vi "RSZVB Set Frequency Conversion Source.vi"(8 "error in (no error)":errorcluster {"code" format="%.0x"}, 10 "Conversion Source (0: Meas. at Source Frequency)":i32(ring) items=["Measurement at Source Frequency", "Measurement at Receiver Frequency"], 11 "VISA session":refnum<visa-resource-name>) -> (0 "error out":errorcluster {"code" format="%.0x"}, 3 "dup VISA session":refnum<visa-resource-name>)   [LabVIEW 2011]
doc: "This VI selects the test setup (internal or external sources) for the frequency converter measurement (with option ZVA-K8, Enhanced Frequency Conversion). \n\n\nNote(s):\n\n(1) This VI is available only on R&S ZVA and ZVT instrument.\n\nRemote-control command(s):\nSENSe<Ch>:FREQuency:CONVersion:DEVice:MODE RILI | RILE"
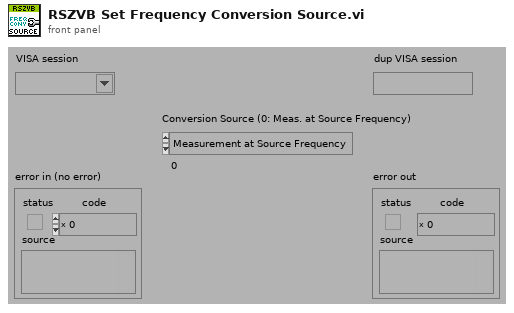
[diagram p1: front panel]
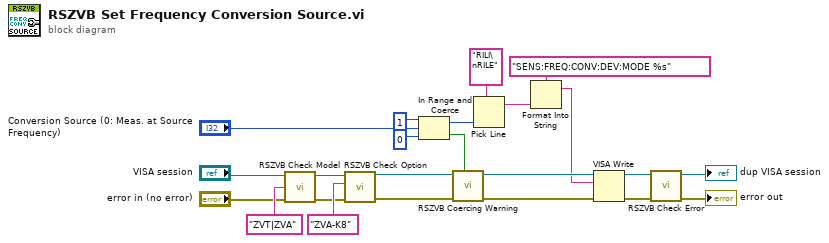
[diagram p0: block diagram]
diagram:
  n1 = call "RSZVB Check Model.vi"("error in (no error)"="error in (no error)", "Model"="ZVT|ZVA" ("Options"), "VISA session"="VISA session") -> ("error out"=w20:errorcluster, "dup VISA session"=w21:refnum<visa-resource-name>)  [unwired: 7 in]
  n2 = call "RSZVB Check Option.vi"("error in (no error)"=w20, "Options"="ZVA-K8", "VISA session"=w21) -> ("error out"=w7:errorcluster, "dup VISA session"=w6:refnum<visa-resource-name>)  [unwired: 7 in]
  n3 = In Range and Coerce(upper limit=1, x="Conversion Source (0: Meas. at Source Frequency)", lower limit=0) -> (coerced(x)=w9:i32, In Range?=w12:bool)
  n4 = call "RSZVB Coercing Warning.vi"("In Range?"=w12, "error in (no error)"=w7, "VISA session"=w6) -> ("error out"=w15:errorcluster, "dup VISA session"=w16:refnum<visa-resource-name>)  [unwired: 7 in]
  n5 = Pick Line(multi-line string="RILI\nRILE", line index=w9) -> (output string=w8:string)  [unwired: 1 in]
  n6 = Format Into String(format string="SENS:FREQ:CONV:DEV:MODE %s", w8) -> (resulting string=w11:string)  [unwired: 2 in, 1 out]
  n7 = VISA Write(VISA resource name=w16, write buffer=w11, error in (no error)=w15) -> (VISA resource name out=w13:refnum<visa-resource-name>, error out=w14:errorcluster)  [unwired: 1 out]
  n8 = call "RSZVB Check Error.vi"("error in (no error)"=w14, "VISA session"=w13) -> ("error out"=→"error out":errorcluster, "dup VISA session"=→"dup VISA session":refnum<visa-resource-name>)  [unwired: 8 in]
